vi "Initialize.vi"(8 "error in (no error)":errorcluster, 11 "Motor Base in":refnum<class "Motor Base.lvclass">) -> (0 "error out":errorcluster, 3 "Motor Base out":refnum<class "Motor Base.lvclass">)   [LabVIEW 2016, in "Motor Base.lvlib" / "Motor Base.lvclass"]
uses:
  Motor Base.lvclass
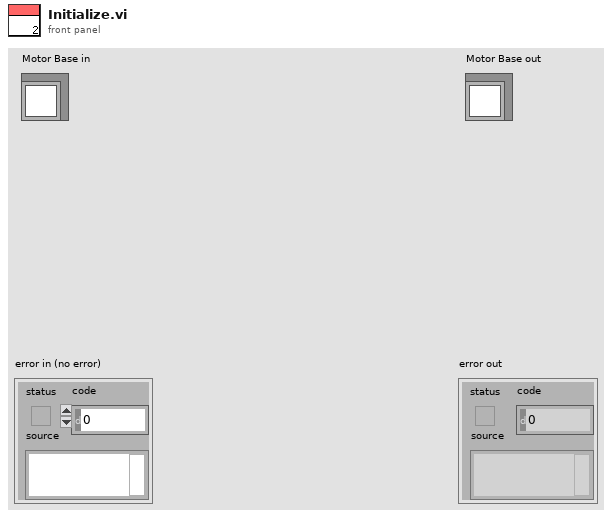
[diagram p1: front panel]
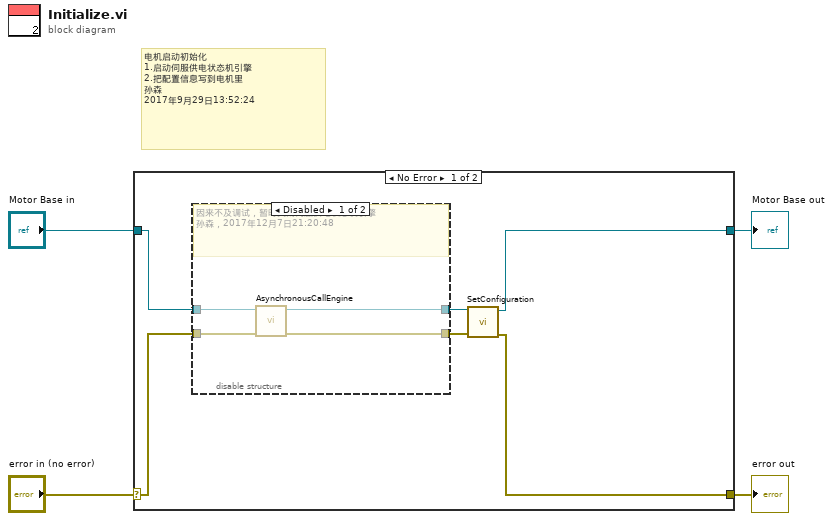
[diagram p0: block diagram]
diagram:
  # "电机启动初始化\n1.启动伺服供电状态机引擎\n2.把配置信息写到电机里\n孙森\n2017年9月29日13:52:24"
  n1 = case shown="No Error" "error in (no error)" {
    selector: "error in (no error)" -> [w9 w18]
    tunnel: [w6 w18] -> w3
    tunnel: [w5 w17] -> w1
    tunnel: "Motor Base in" -> [w10 w17]
    frame No Error {
      n2 = disable-structure shown="Disabled" {
        disable-tunnel: w10 -> [w14 w16]
        disable-tunnel: w9 -> [w13 w15]
        disable-tunnel: [w12 w16] -> w8
        disable-tunnel: [w11 w15] -> w7
        frame Disabled {
          # "因来不及调试，暂时关闭伺服供电状态机引擎\n孙森，2017年12月7日21:20:48"
          n3 = call-dynamic "AsynchronousCallEngine"("error in (no error)"=w13, "Motor Base in"=w14) -> ("error out"=w11:errorcluster, "Motor Base out"=w12:refnum<class "Motor Base.lvclass">)  [unwired: 8 in]
        }
        frame Enabled {
        }
      }
      n4 = call-dynamic "SetConfiguration.vi"("error in (no error)"=w7, "Motor Base in"=w8) -> ("error out"=w6:errorcluster, "Motor Base out"=w5:refnum<class "Motor Base.lvclass">)  [unwired: 8 in]
    }
    frame Error {
    }
  }
  "error out" <- w3
  "Motor Base out" <- w1
